vi "Instruction.vi"(4 "Initialize?":bool, 5 "DI Task":refnum<k21>, 6 "All Flash?":bool, 7 "Touch lines":T2={"Home touch"=0, "Touch 1"=1, "Touch 2"=2, "Touch 3"=3, "Touch 4"=4}, 8 "Instruction duration":dbl, 9 "brightness":i16 caption="Brightness", 10 "Target":i16, 11 "DO Task":refnum<k21>="BlueSimple_DO_All") -> (0 "Last trial successful?":bool, 3 "Go to stage":T1(ring))   [LabVIEW 2010]
doc: "This vi lights and unlights a target light, or all 4 targets if all flash is selected. The lights are lit when the \"initialize\" pane is run, and the other pane, when called, checks to see if the desired lighting time has elapsed--if so, it turns the lights off.\n\nOne thing to note is that this vi runs only once when called. In order to use it, you have to put it inside a loop, so that it repeatedly checks the time."
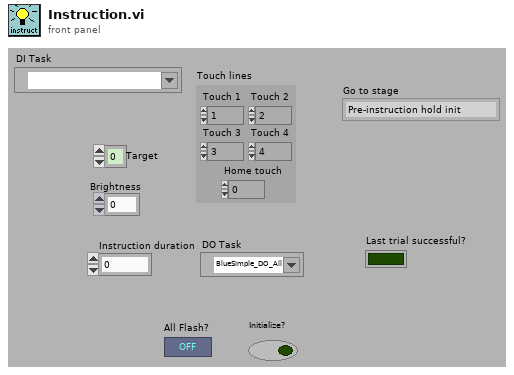
[diagram p1: front panel]
types:
  T1 = enum16{"Pre-instruction hold init", "Pre-instruction hold", "Instruction init", "Instruction", "Post-instruction hold init", "Post-instruction hold", "Target capture init", "Target capture", "Target hold init", "Target hold", "Reward stage", "Intertrial"}
  T2 = cluster{"Home touch":i16, "Touch 1":i16, "Touch 2":i16, "Touch 3":i16, "Touch 4":i16}
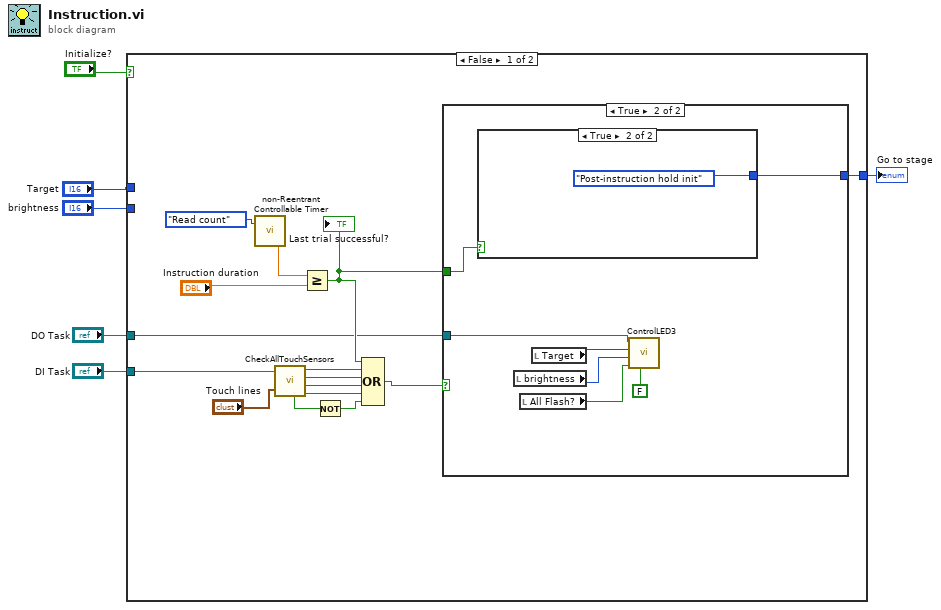
[diagram p0: block diagram]
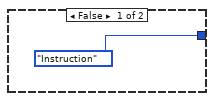
[diagram p2: hidden frame]
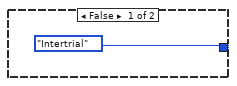
[diagram p3: hidden frame]
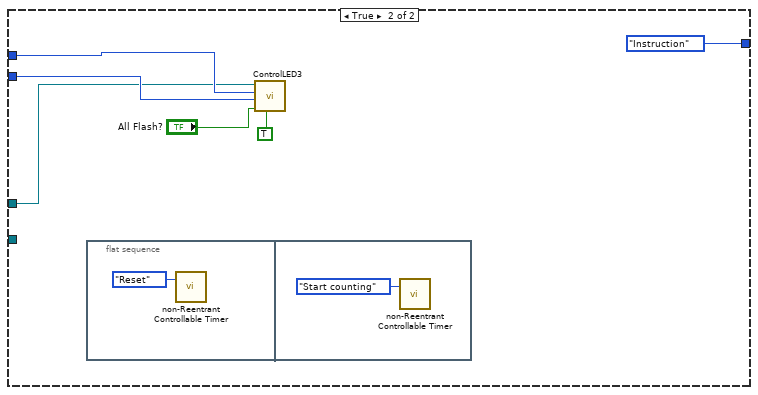
[diagram p4: hidden frame]
diagram:
  n1 = case shown="False" "Initialize?" {
    tunnel: [w21 T1."Instruction" ("Current stage")] -> w3
    tunnel: "Target" -> [_ w35]
    tunnel: "brightness" -> [_ w37]
    tunnel: "DO Task" -> [w8 w32]
    tunnel: "DI Task" -> [w7 _]
    frame False {
      n2 = call "non-Reentrant Controllable Timer.vi"("Enum"=enum16{"Start counting", "Read count", "Reset"}."Read count") -> ("Time out"=w20:dbl)  [unwired: 1 in]
      n3 = call "CheckAllTouchSensors.vi"("Touch sensor lines"="Touch lines", "DI Task"=w7) -> ("TS 4"=w17:bool, "TS 3"=w16:bool, "TS 2"=w15:bool, "TS 1"=w14:bool, "Home?"=w18:bool)
      n4 = Greater Or Equal?(x=w20, y="Instruction duration") -> (x >= y?=w10:bool)
      "Last trial successful?" <- w10
      n5 = Not(x=w18) -> (.not. x?=w19:bool)
      n6 = Compound Arithmetic op=OR(w10, w14, w15, w16, w17, w19) -> (w9:bool)
      n7 = case shown="True" w9 {
        tunnel: [T1."Instruction" ("Current stage") w29] -> w21
        tunnel: w10 -> [_ w28]
        tunnel: w8 -> [_ w23]
        frame False {
        }
        frame True {
          n8 = case shown="True" w28 {
            tunnel: [T1."Intertrial" ("Current stage") T1."Post-instruction hold init" ("Current stage")] -> w29
            frame False {
            }
            frame True {
            }
          }
          n9 = local read "brightness"() -> (w27:i16)
          n10 = local read "All Flash?"() -> (w24:bool)
          n11 = local read "Target"() -> (w26:i16)
          n12 = call "ControlLED3.vi"("On?"=FALSE ("Line state"), "All flash?"=w24, "Brightness"=w27, "Target"=w26, "DO Task"=w23) -> ()  [unwired: 6 in]
        }
      }
    }
    frame True {
      n13 = flat-sequence {
        frame #0 {
          n14 = call "non-Reentrant Controllable Timer.vi"("Enum"=enum16{"Start counting", "Read count", "Reset"}."Reset") -> ()  [unwired: 1 in, 1 out]
        }
        frame #1 {
          n15 = call "non-Reentrant Controllable Timer.vi"("Enum"=enum16{"Start counting", "Read count", "Reset"}."Start counting") -> ()  [unwired: 1 in, 1 out]
        }
      }
      n16 = call "ControlLED3.vi"("On?"=TRUE ("Line state"), "All flash?"="All Flash?", "Brightness"=w37, "Target"=w35, "DO Task"=w32) -> ()  [unwired: 6 in]
    }
  }
  "Go to stage" <- w3
